vi "Return Adapter Message.vi"(8 "error in (no error)":errorcluster, 11 "ReturnMessageAdapter In":refnum<class "ReturnMessageAdapter.lvclass">) -> (0 "error out":errorcluster)   [LabVIEW 2018, in "MVA Framework.lvlib" / "ReturnMessageAdapter.lvclass"]
doc: "返回适配器消息"
uses:
  ReturnMessageAdapter.lvclass
  <vilib>/ActorFramework/Message Enqueuer/Message Enqueuer.lvclass
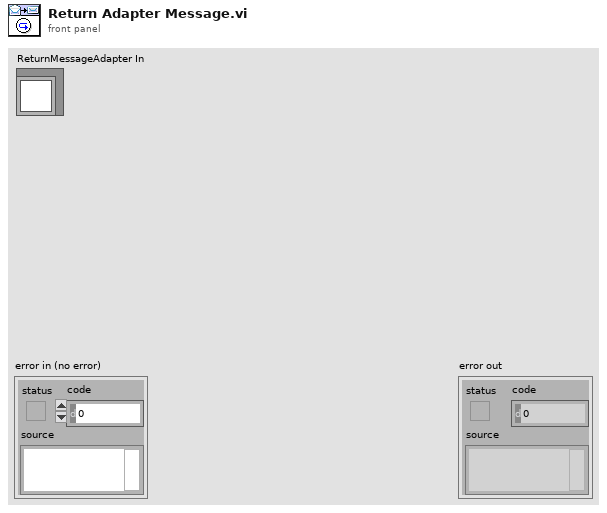
[diagram p1: front panel]
types:
  T1 = typedef "Actor Framework.lvlib/Message Enqueuer.lvclass/Message Priority.ctl" = enum16{"Low", "Normal", "High"}
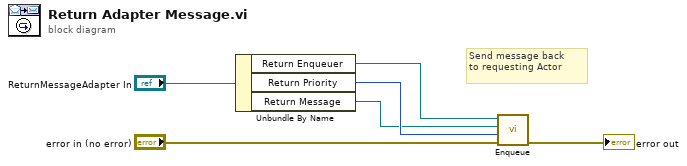
[diagram p0: block diagram]
diagram:
  # "Send message back\nto requesting Actor"
  n1 = Unbundle By Name("ReturnMessageAdapter In") -> ("Return Enqueuer"=w4:refnum<class "Message Enqueuer.lvclass">, "Return Priority"=w2:T1, "Return Message"=w1:refnum<class "Message.lvclass">)
  n2 = call <vilib>:"Enqueue.vi"("error in (no error)"="error in (no error)", "Message Priority (Normal)"=w2, "Message"=w1, "Message Enqueuer in"=w4) -> ("error out"=→"error out":errorcluster)  [unwired: 6 in, 1 out]
